vi "Add File to Lib.vi"(8 "error in (no error)":errorcluster, 10 "File Path":path, 11 "Library in":refnum<vi>) -> (0 "error out":errorcluster, 2 "File Ref":refnum<vi>, 3 "Library out":refnum<vi>)   [LabVIEW 2019, in "VI Scripting Tools.lvlib"]
uses:
  VI Scripting Tools.lvlib
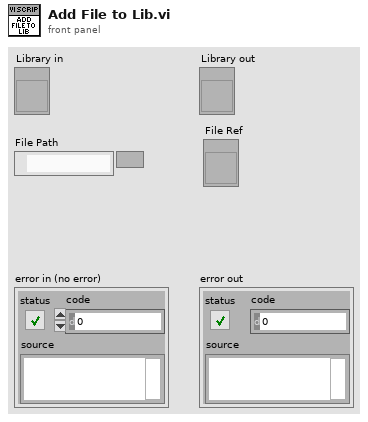
[diagram p1: front panel]
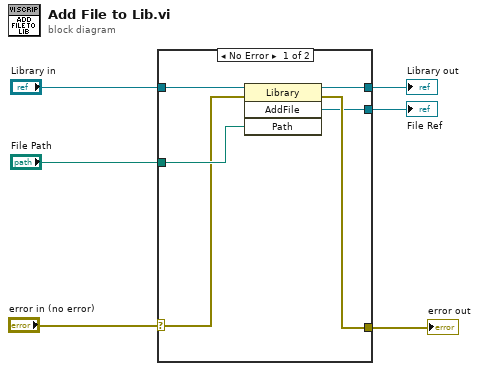
[diagram p0: block diagram]
diagram:
  n1 = case shown="No Error" "error in (no error)" {
    selector: "error in (no error)" -> [w7 w14]
    tunnel: "Library in" -> [w12 w13]
    tunnel: [w11 w13] -> w5
    tunnel: "File Path" -> [w10 _]
    tunnel: [w9 w14] -> w3
    tunnel: [w8 _] -> w2
    frame No Error {
      n2 = invoke class="Library" method="AddFile"(reference=w12, error in=w7, "Path"=w10) -> (reference out=w11:refnum<vi>, error out=w9:errorcluster, "AddFile"=w8:refnum<vi>)  [unwired: 1 in, 1 out]
    }
    frame Error {
    }
  }
  "Library out" <- w5
  "error out" <- w3
  "File Ref" <- w2
